vi "Sub_predictor_v2(SubVI).vi"(6 "predicted step":dbl=0.04 format="%#_13g", 8 "Sim_running":bool, 9 "q_i":dbl[](array[numeric]), 11 "t [s]":dbl) -> (0 "Euler Angles Table [deg]":dbl[](array[numeric]), 3 "Euler Angles Table_pred [deg]":dbl[](array[numeric]))   [LabVIEW 2017]
uses:
  <vilib>/Analysis/coordinate.llb/Euler Rotation Order.ctl
  <vilib>/Analysis/7linalg.llb/Real Transpose Matrix.vi
  <vilib>/Analysis/baseanly.llb/Real A x B.vi
  <vilib>/Analysis/_algsub.llb/Real PseudoInverse Matrix.vi
  <vilib>/Analysis/Matrix/Numeric/Conversions/Array To Matrix - RA2.vi
  <vilib>/Analysis/Matrix/Numeric/Conversions/Array To Matrix - RA.vi
  <vilib>/Analysis/Matrix/Numeric/Conversions/Matrix To Array - RM.vi
  <vilib>/Analysis/Matrix/NI_Matrix.lvlib
  <vilib>/Analysis/NI_AALPro.lvlib
  <vilib>/Analysis/NI_AALBase.lvlib
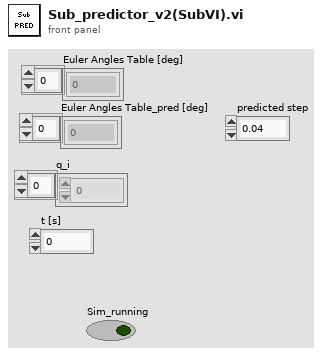
[diagram p1: front panel]
types:
  T1 = typedef "NI_AALPro.lvlib/Euler Rotation Order.ctl" = u16
  T2 = typedef "NI_Matrix.lvlib/RealMatrix.ctl" = dbl[][]
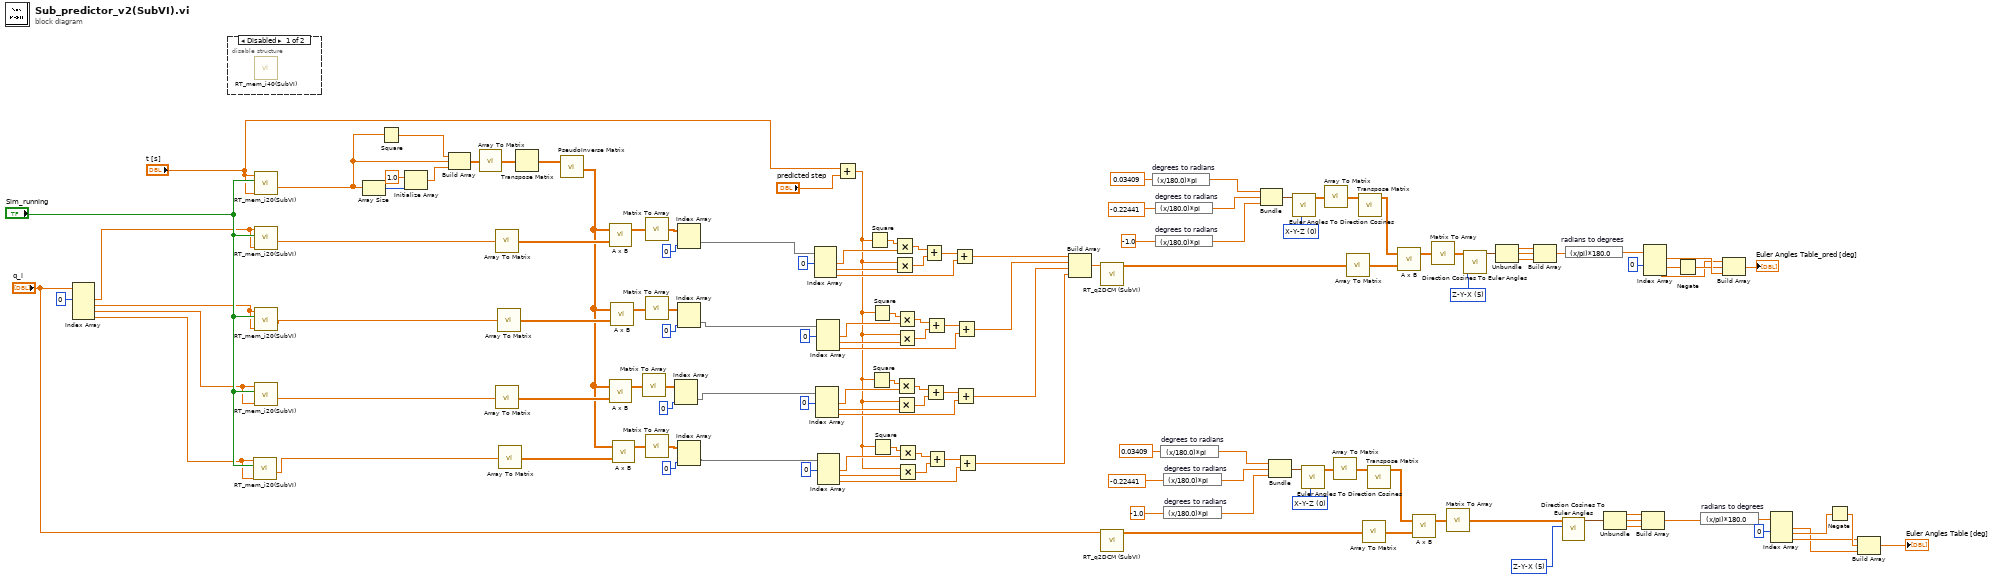
[diagram p0: block diagram]
diagram:
  w15 = T1 0 items=["X-Y-Z", "X-Z-Y", "Y-X-Z", "Y-Z-X", "Z-X-Y", "Z-Y-X", "X-Y-X", "X-Z-X", "Y-X-Y", "Y-Z-Y", "Z-X-Z", "Z-Y-Z"] ("rotation order")
  w30 = T1 0 items=["X-Y-Z", "X-Z-Y", "Y-X-Z", "Y-Z-X", "Z-X-Y", "Z-Y-X", "X-Y-X", "X-Z-X", "Y-X-Y", "Y-Z-Y", "Z-X-Z", "Z-Y-Z"] ("rotation order")
  w33 = T1 5 items=["X-Y-Z", "X-Z-Y", "Y-X-Z", "Y-Z-X", "Z-X-Y", "Z-Y-X", "X-Y-X", "X-Z-X", "Y-X-Y", "Y-Z-Y", "Z-X-Z", "Z-Y-Z"] ("rotation order")
  w57 = T1 5 items=["X-Y-Z", "X-Z-Y", "Y-X-Z", "Y-Z-X", "Z-X-Y", "Z-Y-X", "X-Y-X", "X-Z-X", "Y-X-Y", "Y-Z-Y", "Z-X-Z", "Z-Y-Z"] ("rotation order")
  n1 = Index Array(array="q_i", index #1=0 ("index")) -> (element #1=w106:dbl, element #2=w105:dbl, element #3=w104:dbl, element #4=w103:dbl)  [unwired: 3 in]
  n2 = disable-structure shown="Disabled" {
    frame Disabled {
      n3 = call "RT_mem_i40(SubVI).vi"() -> ()  [unwired: 11 in, 1 out]
    }
    frame Enabled {
    }
  }
  n4 = call "RT_mem_i20(SubVI).vi"("Ini_val"=w103, "start"="Sim_running", "In"=w103) -> ("in_vec"=w109:dbl[])  [unwired: 7 in, 1 out]
  n5 = call "RT_mem_i20(SubVI).vi"("Ini_val"="t [s]", "start"="Sim_running", "In"="t [s]") -> ("in_vec"=w117:dbl[])  [unwired: 7 in, 1 out]
  n6 = call "RT_mem_i20(SubVI).vi"("Ini_val"=w106, "start"="Sim_running", "In"=w106) -> ("in_vec"=w129:dbl[])  [unwired: 7 in, 1 out]
  n7 = call "RT_mem_i20(SubVI).vi"("Ini_val"=w105, "start"="Sim_running", "In"=w105) -> ("in_vec"=w126:dbl[])  [unwired: 7 in, 1 out]
  n8 = call "RT_mem_i20(SubVI).vi"("Ini_val"=w104, "start"="Sim_running", "In"=w104) -> ("in_vec"=w130:dbl[])  [unwired: 7 in, 1 out]
  n9 = Array Size(array=w117) -> (size(s)=w114:i32)
  n10 = Square(x=w117) -> (x^2=w116:dbl[])
  n11 = Initialize Array(1.0 ("element"), w114) -> (w118:dbl[])
  n12 = Build Array(w116, w117, w118) -> (w120:dbl[][])
  n13 = call-poly <vilib>:"Array To Matrix.vi"("Real 2D Array"=w120) -> ("Real Matrix"=w119:T2)
  n14 = call-poly <vilib>:"Array To Matrix.vi"("Real 1D Array"=w129) -> ("Real Matrix (Column Vector)"=w127:T2)
  n15 = call-poly <vilib>:"Array To Matrix.vi"("Real 1D Array"=w130) -> ("Real Matrix (Column Vector)"=w128:T2)
  n16 = call-poly <vilib>:"Array To Matrix.vi"("Real 1D Array"=w126) -> ("Real Matrix (Column Vector)"=w122:T2)
  n17 = call-poly <vilib>:"Array To Matrix.vi"("Real 1D Array"=w109) -> ("Real Matrix (Column Vector)"=w113:T2)
  n18 = Transpose Matrix(1:w119) -> (0:w121:T2)
  n19 = call-poly <vilib>:"PseudoInverse Matrix.vi"("Input Matrix"=w121) -> ("PseudoInverse Matrix"=w108:T2)  [unwired: 1 in, 1 out]
  n20 = call-poly <vilib>:"A x B.vi"("B"=w127, "A"=w108) -> ("A x B"=w135:T2)  [unwired: 1 out]
  n21 = call-poly <vilib>:"A x B.vi"("B"=w128, "A"=w108) -> ("A x B"=w136:T2)  [unwired: 1 out]
  n22 = call-poly <vilib>:"A x B.vi"("B"=w122, "A"=w108) -> ("A x B"=w125:T2)  [unwired: 1 out]
  n23 = call-poly <vilib>:"A x B.vi"("B"=w113, "A"=w108) -> ("A x B"=w110:T2)  [unwired: 1 out]
  n24 = call-poly <vilib>:"Matrix To Array.vi"("Real Matrix"=w136) -> ("Real 2D Array"=w133:dbl[][])
  n25 = call-poly <vilib>:"Matrix To Array.vi"("Real Matrix"=w135) -> ("Real 2D Array"=w132:dbl[][])
  n26 = call-poly <vilib>:"Matrix To Array.vi"("Real Matrix"=w125) -> ("Real 2D Array"=w123:dbl[][])
  n27 = call-poly <vilib>:"Matrix To Array.vi"("Real Matrix"=w110) -> ("Real 2D Array"=w112:dbl[][])
  n28 = Index Array(array=w133, index (col)=0 ("index (row)")) -> (element=w65:dbl[])  [unwired: 1 in]
  n29 = Index Array(array=w132, index (col)=0 ("index (row)")) -> (element=w92:dbl[])  [unwired: 1 in]
  n30 = Index Array(array=w123, index (col)=0 ("index (row)")) -> (element=w66:dbl[])  [unwired: 1 in]
  n31 = Index Array(array=w112, index (col)=0 ("index (row)")) -> (element=w64:dbl[])  [unwired: 1 in]
  n32 = Index Array(array=w92, index #1=0 ("index")) -> (element #1=w95:dbl, element #2=w97:dbl, element #3=w100:dbl)  [unwired: 2 in]
  n33 = Index Array(array=w65, index #1=0 ("index")) -> (element #1=w77:dbl, element #2=w79:dbl, element #3=w82:dbl)  [unwired: 2 in]
  n34 = Index Array(array=w66, index #1=0 ("index")) -> (element #1=w88:dbl, element #2=w86:dbl, element #3=w83:dbl)  [unwired: 2 in]
  n35 = Index Array(array=w64, index #1=0 ("index")) -> (element #1=w72:dbl, element #2=w70:dbl, element #3=w67:dbl)  [unwired: 2 in]
  n36 = Add(x="t [s]", y="predicted step") -> (x+y=w63:dbl)
  n37 = Square(x=w63) -> (x^2=w94:dbl)
  n38 = Square(x=w63) -> (x^2=w76:dbl)
  n39 = Square(x=w63) -> (x^2=w89:dbl)
  n40 = Square(x=w63) -> (x^2=w73:dbl)
  n41 = Multiply(x=w94, y=w95) -> (x*y=w96:dbl)
  n42 = Multiply(x=w63, y=w97) -> (x*y=w98:dbl)
  n43 = Multiply(x=w76, y=w77) -> (x*y=w78:dbl)
  n44 = Multiply(x=w63, y=w79) -> (x*y=w80:dbl)
  n45 = Multiply(x=w89, y=w88) -> (x*y=w87:dbl)
  n46 = Multiply(x=w63, y=w86) -> (x*y=w85:dbl)
  n47 = Multiply(x=w73, y=w72) -> (x*y=w71:dbl)
  n48 = Multiply(x=w63, y=w70) -> (x*y=w69:dbl)
  n49 = Add(x=w96, y=w98) -> (x+y=w99:dbl)
  n50 = Add(x=w78, y=w80) -> (x+y=w81:dbl)
  n51 = Add(x=w87, y=w85) -> (x+y=w84:dbl)
  n52 = Add(x=w71, y=w69) -> (x+y=w68:dbl)
  n53 = Add(x=w99, y=w100) -> (x+y=w62:dbl)
  n54 = Add(x=w81, y=w82) -> (x+y=w60:dbl)
  n55 = Add(x=w84, y=w83) -> (x+y=w61:dbl)
  n56 = Add(x=w68, y=w67) -> (x+y=w59:dbl)
  n57 = Build Array(w62, w61, w60, w59) -> (w58:dbl[])
  n58 = call "RT_q2DCM (SubVI).vi"("Quaternion"=w58) -> ("DCM"=w19:dbl[][])  [unwired: 10 in]
  n59 = call "RT_q2DCM (SubVI).vi"("Quaternion"="q_i") -> ("DCM"=w4:dbl[][])  [unwired: 10 in]
  n60 = expression code="(x/180.0)*pi" "degrees to radians"(0.03409 ("y")) -> (w29:dbl)
  n61 = expression code="(x/180.0)*pi" "degrees to radians"(-0.22441 ("y")) -> (w28:dbl)
  n62 = expression code="(x/180.0)*pi" "degrees to radians"(-1.0 ("y")) -> (w27:dbl)
  n63 = expression code="(x/180.0)*pi" "degrees to radians"(0.03409 ("y")) -> (w14:dbl)
  n64 = expression code="(x/180.0)*pi" "degrees to radians"(-0.22441 ("y")) -> (w13:dbl)
  n65 = expression code="(x/180.0)*pi" "degrees to radians"(-1.0 ("y")) -> (w12:dbl)
  n66 = Bundle("y"=w29, "y"=w28, "y"=w27) -> (w31:cluster{"y":dbl, "y":dbl, "y":dbl})  [unwired: 1 in]
  n67 = Bundle("y"=w14, "y"=w13, "y"=w12) -> (w16:cluster{"y":dbl, "y":dbl, "y":dbl})  [unwired: 1 in]
  n68 = call <vilib>:"Euler Angles To Direction Cosines.vi"("rotation order"=w30, "Euler Angles"=w31) -> ("Direction Cosines"=w23:dbl[][])  [unwired: 8 in, 1 out]
  n69 = call <vilib>:"Euler Angles To Direction Cosines.vi"("rotation order"=w15, "Euler Angles"=w16) -> ("Direction Cosines"=w9:dbl[][])  [unwired: 8 in, 1 out]
  n70 = call-poly <vilib>:"Array To Matrix.vi"("Real 2D Array"=w23) -> ("Real Matrix"=w22:T2)
  n71 = call-poly <vilib>:"Array To Matrix.vi"("Real 2D Array"=w9) -> ("Real Matrix"=w8:T2)
  n72 = call-poly <vilib>:"Array To Matrix.vi"("Real 2D Array"=w19) -> ("Real Matrix"=w21:T2)
  n73 = call-poly <vilib>:"Transpose Matrix.vi"("Input Matrix"=w22) -> ("Matrix Transpose"=w20:T2)  [unwired: 9 in, 1 out]
  n74 = call-poly <vilib>:"Array To Matrix.vi"("Real 2D Array"=w4) -> ("Real Matrix"=w7:T2)
  n75 = call-poly <vilib>:"Transpose Matrix.vi"("Input Matrix"=w8) -> ("Matrix Transpose"=w6:T2)  [unwired: 9 in, 1 out]
  n76 = call-poly <vilib>:"A x B.vi"("B"=w21, "A"=w20) -> ("A x B"=w18:T2)  [unwired: 1 out]
  n77 = call-poly <vilib>:"A x B.vi"("B"=w7, "A"=w6) -> ("A x B"=w5:T2)  [unwired: 1 out]
  n78 = call-poly <vilib>:"Matrix To Array.vi"("Real Matrix"=w18) -> ("Real 2D Array"=w17:dbl[][])
  n79 = call-poly <vilib>:"Matrix To Array.vi"("Real Matrix"=w5) -> ("Real 2D Array"=w3:dbl[][])
  n80 = call <vilib>:"Direction Cosines To Euler Angles.vi"("rotation order"=w57, "Direction Cosines"=w17) -> ("Euler Angles"=w54:cluster{"phi":dbl, "theta":dbl, "psi":dbl})  [unwired: 8 in, 1 out]
  n81 = Unbundle(w54) -> ("phi"=w56:dbl, "theta"=w55:dbl, "psi"=w53:dbl)
  n82 = Build Array(w56, w55, w53) -> (w46:dbl[])
  n83 = call <vilib>:"Direction Cosines To Euler Angles.vi"("rotation order"=w33, "Direction Cosines"=w3) -> ("Euler Angles"=w36:cluster{"phi":dbl, "theta":dbl, "psi":dbl})  [unwired: 8 in, 1 out]
  n84 = expression code="(x/pi)*180.0" "radians to degrees"(w46) -> (w49:dbl[])
  n85 = Unbundle(w36) -> ("phi"=w34:dbl, "theta"=w35:dbl, "psi"=w37:dbl)
  n86 = Build Array(w34, w35, w37) -> (w45:dbl[])
  n87 = Index Array(array=w49, index #1=0 ("index")) -> (element #1=w51:dbl, element #2=w47:dbl, element #3=w1:dbl)  [unwired: 2 in]
  n88 = Negate(x=w47) -> (-x=w48:dbl)
  n89 = expression code="(x/pi)*180.0" "radians to degrees"(w45) -> (w41:dbl[])
  n90 = Build Array(w1, w48, w51) -> (→"Euler Angles Table_pred [deg]":dbl[])
  n91 = Index Array(array=w41, index #1=0 ("index")) -> (element #1=w39:dbl, element #2=w44:dbl, element #3=w42:dbl)  [unwired: 2 in]
  n92 = Negate(x=w44) -> (-x=w43:dbl)
  n93 = Build Array(w42, w43, w39) -> (→"Euler Angles Table [deg]":dbl[])
